vi "myRIO v1.0 Decode Encoder STAT.vi"(11 "ENC.STAT":u8) -> (0 "ENC.CNFG to write":u8, 1 "Signed Overflow?":bool, 2 "Error?":bool, 3 "Counting down?":bool, 5 "Signed Overflow Error?":bool)   [LabVIEW 2021]
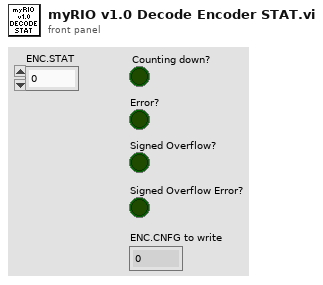
[diagram p1: front panel]
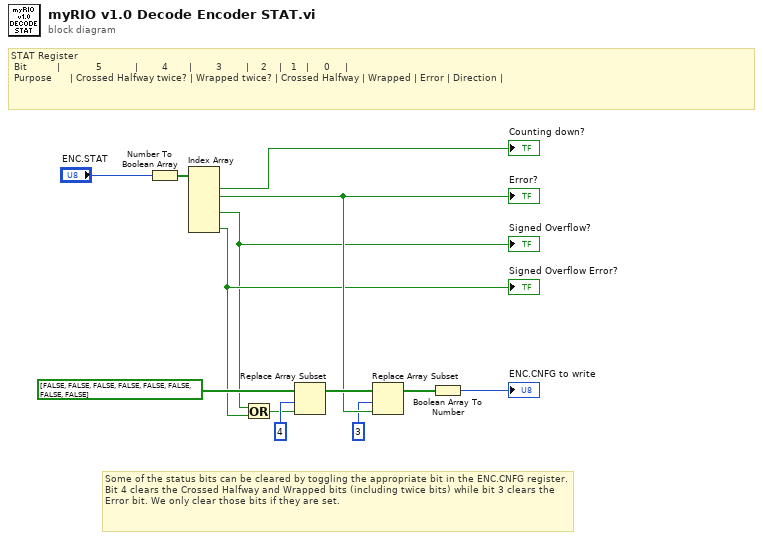
[diagram p0: block diagram]
diagram:
  # "STAT Register\n Bit          |            5           |        4       |        3        |    2    |   1   |     0     |\n Purpose      | Crossed Halfway twice? | Wrapped twice? | Crossed Halfway | Wrapped | Error | Direction |"
  # "Some of the status bits can be cleared by toggling the appropriate bit in the ENC.CNFG register. Bit 4 clears the Crossed Halfway and Wrapped bits (including twice bits) while bit 3 clears the Error bit. We only clear those bits if they are set."
  n1 = Number To Boolean Array(number="ENC.STAT") -> (Boolean array=w12:bool[])
  n2 = Index Array(array=w12) -> (element #1=→"Counting down?":bool, element #2=w8:bool, element #4=w2:bool, element #6=w3:bool)  [unwired: 6 in, 2 out]
  "Error?" <- w8
  "Signed Overflow?" <- w2
  "Signed Overflow Error?" <- w3
  n3 = Or(x=w2, y=w3) -> (x .or. y?=w1:bool)
  n4 = Replace Array Subset(array=bool[] [FALSE, FALSE, FALSE, FALSE, FALSE, FALSE, FALSE, FALSE], new element=w1, index=4) -> (w9:bool[])
  n5 = Replace Array Subset(array=w9, new element=w8, index=3) -> (w5:bool[])
  n6 = Boolean Array To Number(Boolean array=w5) -> (number=→"ENC.CNFG to write":u8)
